vi "Write Open.vi"(8 "error in (no error)":errorcluster, 10 "Open":bool, 11 "dir in":refnum<class "dir.lvclass">) -> (0 "error out":errorcluster, 3 "dir out":refnum<class "dir.lvclass">)   [LabVIEW 2023, in "d7.lvlib" / "dir.lvclass"]
uses:
  dir.lvclass
  dir.lvclass/dir.ctl
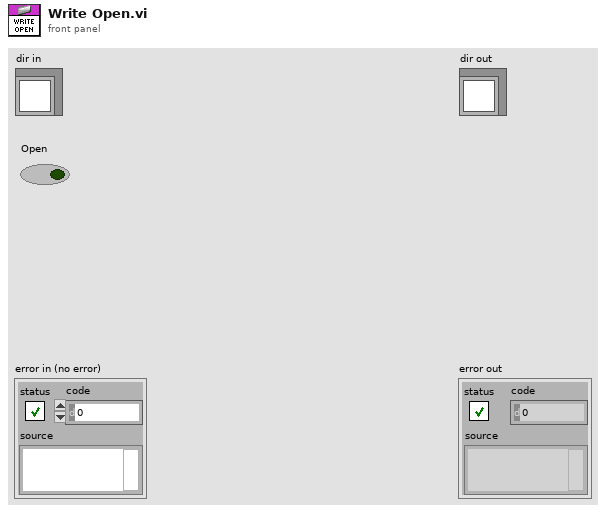
[diagram p1: front panel]
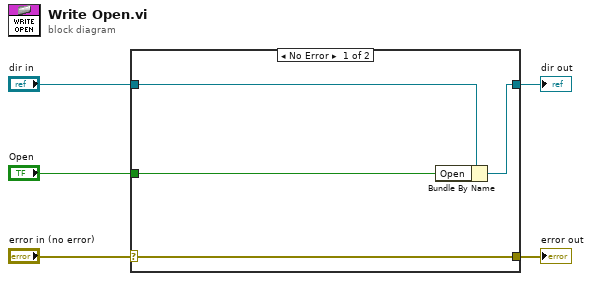
[diagram p0: block diagram]
diagram:
  n1 = case shown="No Error" "error in (no error)" {
    selector: "error in (no error)" -> [w9 w10]
    tunnel: [w9 w10] -> w4
    tunnel: [w7 w11] -> w2
    tunnel: "dir in" -> [w8 w11]
    tunnel: "Open" -> [w6 _]
    frame No Error {
      n2 = Bundle By Name(cluster=w8, "Open"=w6) -> (w7:refnum<class "dir.lvclass">)
    }
    frame Error {
    }
  }
  "error out" <- w4
  "dir out" <- w2
